vi "Wave Filter.vi"(9 "Filter ON":bool, 10 "Value":dbl min=-1.0 max=1.0 step=0.01, 11 "Data In":dbl[](array[numeric])) -> (3 "Data Out":dbl[](array[numeric]))   [LabVIEW 2018]
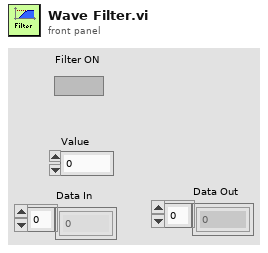
[diagram p1: front panel]
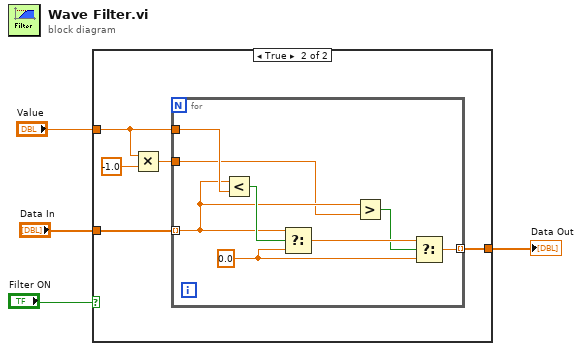
[diagram p0: block diagram]
diagram:
  n1 = case shown="True" "Filter ON" {
    tunnel: "Data In" -> [w5 w10]
    tunnel: "Value" -> [_ w8]
    tunnel: [w5 w6] -> w2
    frame False {
    }
    frame True {
      n2 = Multiply(x=w8, y=-1.0) -> (x*y=w7:dbl)
      n3 = for {
        tunnel: w10 -> [w13] mode=indexing
        tunnel: w8 -> [w18]
        tunnel: w7 -> [w12]
        tunnel: [w14] -> w6 mode=indexing
        w15 = 0.0 ("f")
        n4 = Less?(x=w13, y=w18) -> (x < y?=w17:bool)
        n5 = Select(t=w13, s=w17, f=w15) -> (s? t:f=w16:dbl)
        n6 = Greater?(x=w13, y=w12) -> (0:w11:bool)
        n7 = Select(t=w16, s=w11, f=w15) -> (s? t:f=w14:dbl)
      }
    }
  }
  "Data Out" <- w2
